vi "IFF_WeldMean.vi"() -> ()   [LabVIEW 2014]
uses:
  <vilib>/Utility/file.llb/Write To Spreadsheet File (DBL).vi
panel:
  in  "Save":bool=TRUE
  out "PowMap":dbl[][](graph)
  in  "LowPow":dbl=150.0
  in  "HighPow":dbl=300.0
  in  "Sampling":T1={"Length"=1.0, "NumBins"=20.0, "BinSize"=0.05}
  in  "Y":cluster{"Ymin":dbl, "Ymax":dbl}={"Ymin"=-9.99, "Ymax"=9.99}
  in  "X":cluster{"Xmin":dbl, "Xmax":dbl}={"Xmin"=-9.99, "Xmax"=9.99}
  in  "Rays":u32=100
  in  "PixSize(mm)":dbl=0.1
  out "XY Graph":cluster{cluster{"X":sgl, "Y":sgl}[]}[](graph)=[{[{"X"=5.0, "Y"=2.125}, {"X"=5.0, "Y"=2.625}, {"X"=5.0, "Y"=5.0}, {"X"=2.625, "Y"=5.0}, {"X"=-5.0, "Y"=5.0}, {"X"=-5.0, "Y"=2.625}, {"X"=-5.0, "Y"=-2.125}, {"X"=-5.0, "Y"=-2.625}, {"X"=-5.0, "Y"=-5.0}, {"X"=-2.625, "Y"=-5.0}, {"X"=5.0, "Y"=-5.0}, {"X"=5.0, "Y"=-2.625}, {"X"=5.0, "Y"=2.125}]}, {[{"X"=5.0, "Y"=2.2750006}, {"X"=5.0, "Y"=2.5749998}, {"X"=5.0, "Y"=5.0}, {"X"=2.5749998, "Y"=5.0}, {"X"=-5.0, "Y"=5.0}, {"X"=-5.0, "Y"=2.5749998}, {"X"=-5.0, "Y"=-2.2750006}, {"X"=-5.0, "Y"=-2.5749998}, {"X"=-5.0, "Y"=-5.0}, {"X"=-2.5749998, "Y"=-5.0}, {"X"=5.0, "Y"=-5.0}, {"X"=5.0, "Y"=-2.5749998}, {"X"=5.0, "Y"=2.2750006}]}]
  in  "Thick":dbl=0.05
  in  "Z":dbl=7.625
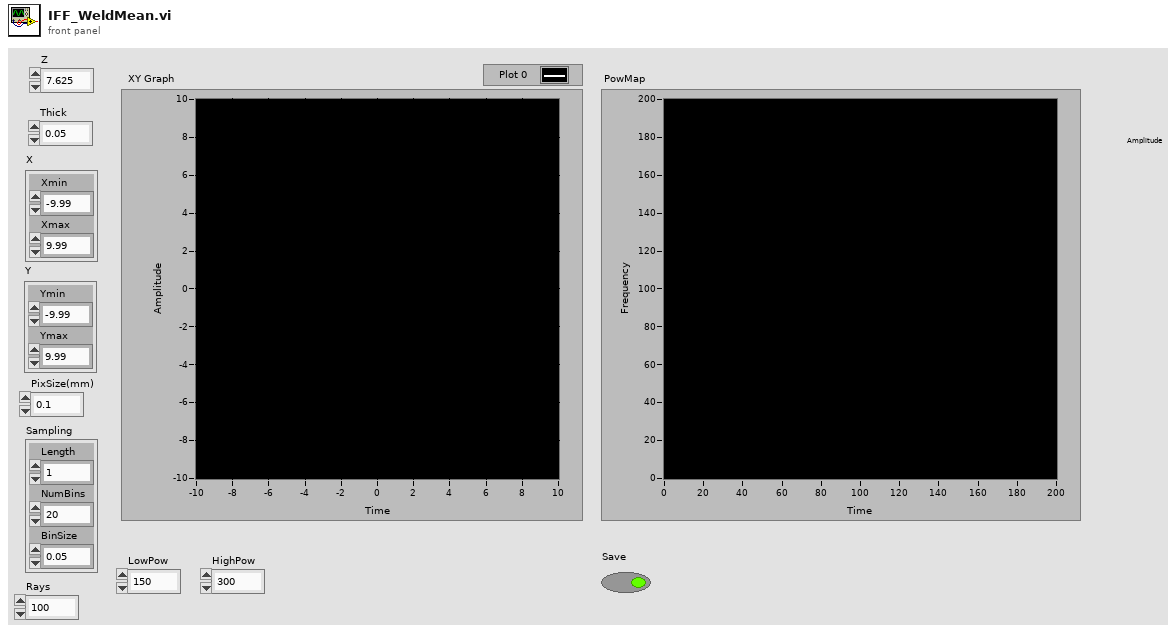
[diagram p1: front panel]
types:
  T1 = cluster{"Length":dbl, "NumBins":dbl, "BinSize":dbl}
  T2 = cluster{"TriVertex":dbl[][], "Normal":dbl[][], "u":dbl[][], "v":dbl[][]}
  T3 = typedef "Poly2DwSlope.ctl" = cluster{"VertexArray":T4[]}
  T4 = typedef "Point2DwSlope.ctl" = cluster{"X":sgl, "Y":sgl, "Slope":dbl}
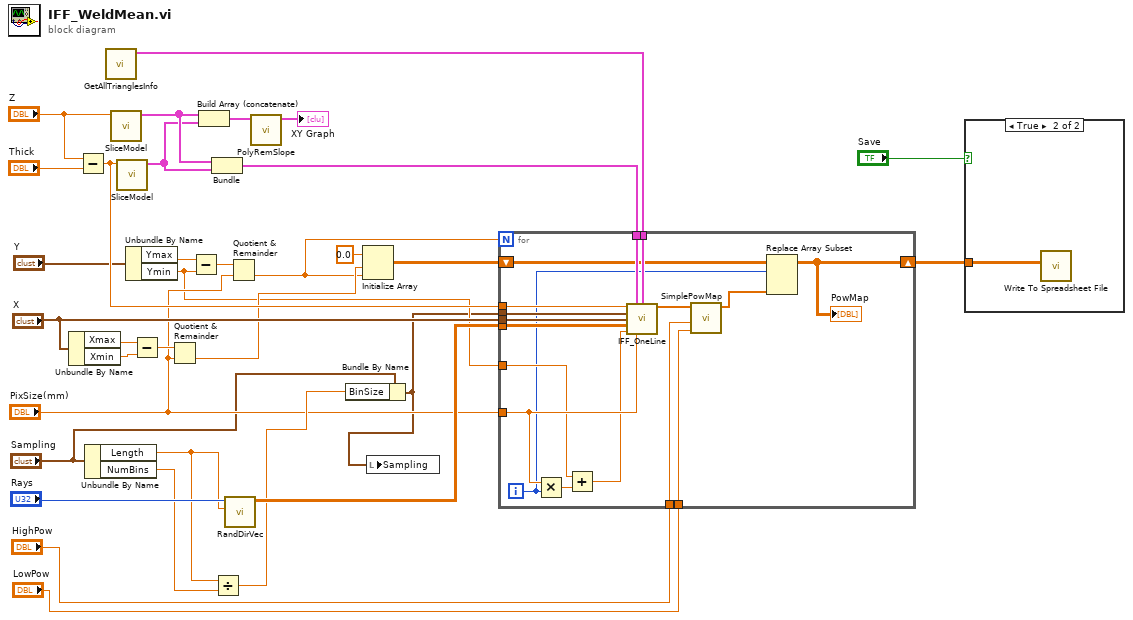
[diagram p0: block diagram]
diagram:
  n1 = Unbundle By Name("X") -> ("Xmax"=w18:dbl, "Xmin"=w19:dbl)
  n2 = Subtract(x="Z", y="Thick") -> (x-y=w29:dbl)
  n3 = Unbundle By Name("Sampling") -> ("Length"=w26:dbl, "NumBins"=w25:dbl)
  n4 = call "GetAllTrianglesInfo.vi"() -> ("TriangleInfo"=w21:T2)  [unwired: 10 in, 1 out]
  n5 = call "SliceModel.vi"("Z"="Z") -> ("Polys"=w23:T3[])  [unwired: 10 in]
  n6 = call "SliceModel.vi"("Z"=w29) -> ("Polys"=w22:T3[])  [unwired: 10 in]
  n7 = Unbundle By Name("Y") -> ("Ymax"=w14:dbl, "Ymin"=w9:dbl)
  n8 = Subtract(x=w18, y=w19) -> (x-y=w17:dbl)
  n9 = Quotient & Remainder(x=w17, y="PixSize(mm)") -> (floor(x/y)=w11:dbl)  [unwired: 1 out]
  n10 = Subtract(x=w14, y=w9) -> (x-y=w15:dbl)
  n11 = Build Array (concatenate)(w23, w22) -> (w31:T3[])
  n12 = Bundle("Polys"=w23, "Polys"=w22) -> (w20:cluster{"Polys":T3[], "Polys":T3[]})  [unwired: 1 in]
  n13 = Divide(x=w26, y=w25) -> (x/y=w24:dbl)
  n14 = call "RandDirVec.vi"("Length"=w26, "Rays"="Rays") -> ("DirVecs"=w27:dbl[][])  [unwired: 9 in]
  n15 = Quotient & Remainder(x=w15, y="PixSize(mm)") -> (floor(x/y)=w8:dbl)  [unwired: 1 out]
  n16 = call "PolyRemSlope.vi"("PolysIn"=w31) -> ("PolysOut"=→"XY Graph":cluster{cluster{"X":sgl, "Y":sgl}[]}[])  [unwired: 10 in]
  n17 = Bundle By Name(cluster="Sampling", "BinSize"=w24) -> (w5:T1)
  n18 = Initialize Array(0.0 ("element"), w11, w8) -> (w7:dbl[][])
  n19 = local write "Sampling"(w5) -> ()
  n20 = for {
    N: w8 -> [_]
    tunnel: w29 -> [w50]
    tunnel: w27 -> [w49]
    tunnel: w5 -> [w48]
    tunnel: w21 -> [w47]
    tunnel: w20 -> [w46]
    tunnel: "X" -> [w45]
    tunnel: "PixSize(mm)" -> [w44]
    tunnel: w9 -> [w42]
    shift-right: [w34] -> w1
    shift-left: w7 -> [w40]
    tunnel: "HighPow" -> [w36]
    tunnel: "LowPow" -> [w35]
    i -> [w39]
    n21 = Multiply(x=w44, y=w39) -> (x*y=w43:dbl)
    n22 = Add(x=w42, y=w43) -> (x+y=w41:dbl)
    n23 = call "IFF_OneLine.vi"("Ztest"=w50, "Slices"=w46, "TriangleInfo"=w47, "Sampling"=w48, "X"=w45, "DirVecs"=w49, "Y"=w41, "PixSize(mm)"=w44) -> ("LineOut"=w38:dbl[])  [unwired: 7 in]
    n24 = call "SimplePowMap.vi"("Low"=w35, "High"=w36, "LineOut"=w38) -> ("Mapped"=w37:dbl[])  [unwired: 8 in]
    n25 = Replace Array Subset(array=w40, new element=w37, index (row)=w39) -> (w34:dbl[][])  [unwired: 1 in]
    "PowMap" <- w34
  }
  n26 = case shown="True" "Save" {
    tunnel: w1 -> [_ w51]
    frame False {
    }
    frame True {
      n27 = call-poly <vilib>:"Write To Spreadsheet File.vi"("2D data"=w51) -> ()  [unwired: 7 in, 1 out]
    }
  }
